vi "Is Changed.vi"(10 "error in (no error)":errorcluster, 11 "Config Manager in":refnum<class "Config Manager.lvclass">) -> (2 "error out":errorcluster, 3 "Changed":bool)   [LabVIEW 2020, in "CDM-Config.lvlib" / "Config Manager.lvclass"]
uses:
  Config Manager.lvclass
  Config Manager.lvclass/Config Manager.ctl
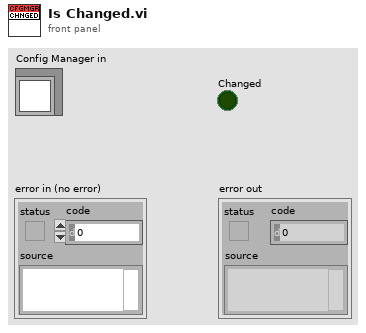
[diagram p1: front panel]
types:
  T1 = typedef "CDM-Config.lvlib/Config Manager.lvclass/Ref Data.ctl" = cluster{"Elements":refnum<class "Config Element.lvclass">[], "Hierarchy Map":map{string[], i32}, "Element Map":map{refnum<class "Config Element.lvclass">, i32}, "Changed":bool[]}
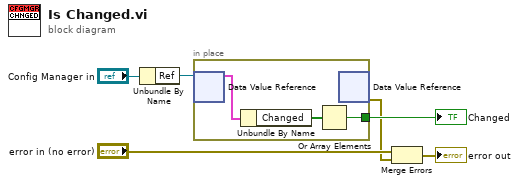
[diagram p0: block diagram]
diagram:
  n1 = Unbundle By Name("Config Manager in") -> ("Ref"=w5:refnum<data-value>)
  n2 = in-place {
    in-place-border: [w7] -> w3
    n3 = in-place-dvr #1(w5) -> (w9:T1)  [unwired: 1 out]
    n4 = Unbundle By Name(w9) -> ("Changed"=w8:bool[])
    n5 = Or Array Elements(Boolean array=w8) -> (logical OR=w7:bool)
    n6 = in-place-dvr #1() -> (w1:errorcluster)  [unwired: 1 in, 1 out]
  }
  "Changed" <- w3
  n7 = Merge Errors("error in (no error)", w1) -> (→"error out":errorcluster)
